vi "Get IDs or Error.vi"(0 "IRegisteredHandler in":refnum<class "IRegisteredHandler.lvclass">, 11 "error in (no error)":errorcluster) -> (4 "IRegisteredHandler out":refnum<class "IRegisteredHandler.lvclass">, 6 "Request ID":u64, 8 "Registration ID":u64, 10 "ErrorOrSuccess":refnum<class "ErrorOrSuccess.lvclass">, 15 "error out":errorcluster)   [LabVIEW 2020, in "wamplv.lvlib" / "IRegisteredHandler.lvclass"]
uses:
  IRegisteredHandler.lvclass
  Message loop classes/ErrorOrSuccess/ErrorOrSuccess.lvclass
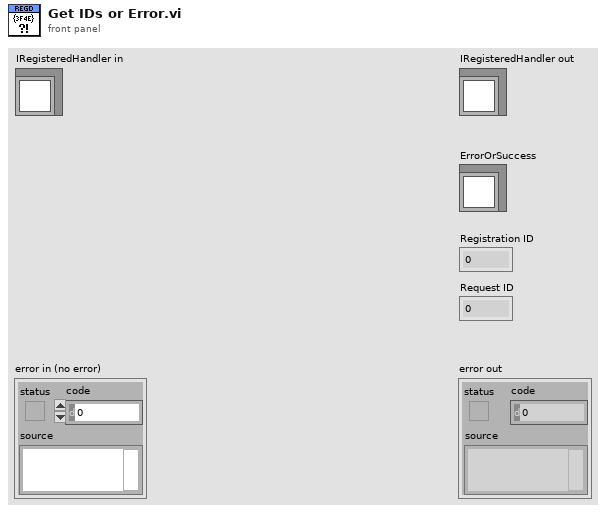
[diagram p1: front panel]
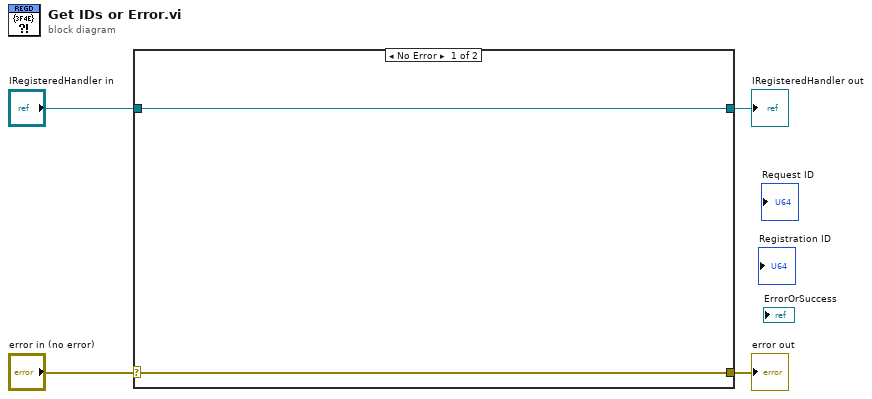
[diagram p0: block diagram]
diagram:
  n1 = case shown="No Error" "error in (no error)" {
    selector: "error in (no error)" -> [w5 w8]
    tunnel: [w5 w8] -> w3
    tunnel: [w6 w7] -> w1
    tunnel: "IRegisteredHandler in" -> [w6 w7]
    frame No Error {
    }
    frame Error {
    }
  }
  "error out" <- w3
  "IRegisteredHandler out" <- w1
